vi "OAT Tachless Connect Trace.vi"(10 "Pop Pos":cluster{i32, i32}, 11 "Tracks Ref":refnum<vi>) -> ()   [LabVIEW 2017, in "SoundVib_Tachless.lvlib"]
uses:
  <vilib>/addons/Sound and Vibration/Order Analysis/Tachless/SoundVib_Tachless.lvlib
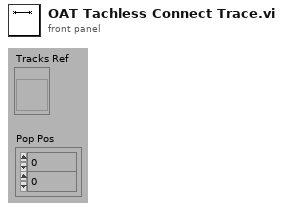
[diagram p1: front panel]
types:
  T1 = cluster{"Name":string, "Color":u32, "Style":u8, "Point Style":u8, "Name Visible":bool, "Allow Drag":bool, "Lock Style":u32, "Plot":u32, "Index":i32, "Position":cluster{"X":dbl, "Y":dbl}}[]
  T2 = cluster{"Name":string, "Color":u32, "Hair Style":u8, "Point Style":u8, "Name Visible":bool, "Trackable":bool, "Lock Style":u32, "Plot Number":u32, "Marker Index":i32, "Location":cluster{"X":dbl, "Y":dbl}}[]
  T3 = cluster{"Name":string, "Color":u32, "Hair Style":u8, "Point Style":u8, "Name Visible":bool, "Trackable":bool, "Lock Style":u32, "Plot Number":u32, "Marker Index":i32, "Location":cluster{"X":dbl, "Y":dbl}}
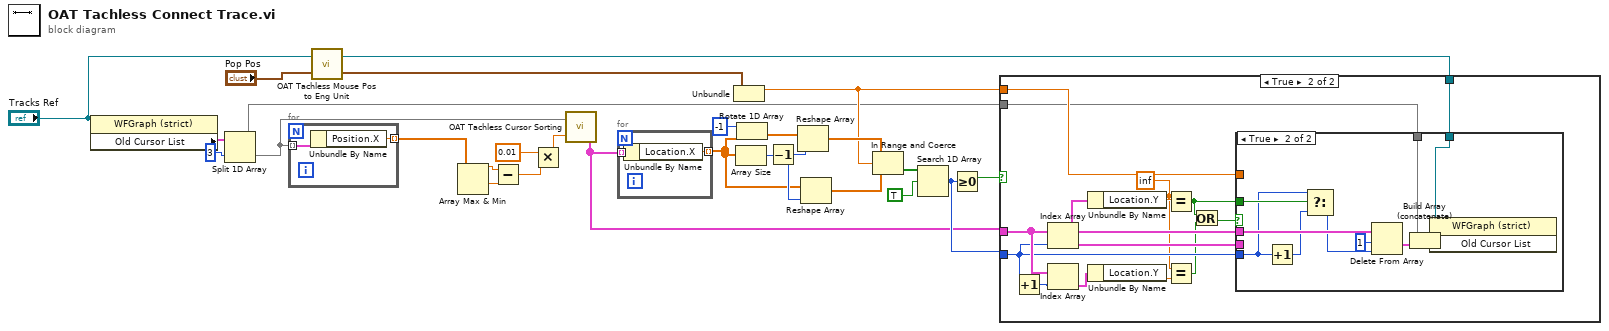
[diagram p0: block diagram]
diagram:
  n1 = property on="Property Node" class="WFGraph (strict)"(reference="Tracks Ref") -> ("Old Cursor List"=w25:T1)  [unwired: 1 in, 2 out]
  n2 = Split 1D Array(array=w25, index=3 ("Array Index")) -> (first subarray=w3:T1, second subarray=w2:T1)
  n3 = for {
    tunnel: w2 -> [w28] mode=indexing
    tunnel: [w27] -> w5 mode=indexing
    n4 = Unbundle By Name(w28) -> ("Position.X"=w27:dbl)
  }
  n5 = call <vilib>:"OAT Tachless Mouse Pos to Eng Unit.vi"("Pop Pos"="Pop Pos", "Tracks ref"="Tracks Ref") -> ("Control Point"=w17:cluster{dbl, dbl})  [unwired: 1 in]
  n6 = Array Max & Min(array=w5) -> (max value=w10:dbl, min value=w9:dbl)  [unwired: 2 out]
  n7 = Subtract(x=w10, y=w9) -> (x-y=w8:dbl)
  n8 = Multiply(x=0.01, y=w8) -> (x*y=w6:dbl)
  n9 = call <vilib>:"OAT Tachless Cursor Sorting.vi"("Numeric"=w6, "Array"=w2) -> ("Array 2"=w1:T2)
  n10 = for {
    tunnel: w1 -> [w30] mode=indexing
    tunnel: [w29] -> w4 mode=indexing
    n11 = Unbundle By Name(w30) -> ("Location.X"=w29:dbl)
  }
  n12 = Unbundle(w17) -> (w14:dbl)  [unwired: 1 out]
  n13 = Array Size(array=w4) -> (size(s)=w21:i32)
  n14 = Rotate 1D Array(1:w4, 2:-1 ("n")) -> (0:w22:dbl[])
  n15 = Decrement(x=w21) -> (x-1=w20:i32)
  n16 = Reshape Array(w22, w20) -> (w19:dbl[])
  n17 = Reshape Array(w4, w20) -> (w18:dbl[])
  n18 = In Range and Coerce(upper limit=w19, x=w14, lower limit=w18) -> (In Range?=w16:bool[])  [unwired: 1 out]
  n19 = Search 1D Array(1D array=w16, element=TRUE) -> (index of element=w13:i32)  [unwired: 1 in]
  n20 = Greater Or Equal To 0?(x=w13) -> (x >= 0?=w12:bool)
  n21 = case shown="True" w12 {
    tunnel: w13 -> [_ w39]
    tunnel: w1 -> [_ w40]
    tunnel: w14 -> [_ w43]
    tunnel: "Tracks Ref" -> [_ w42]
    tunnel: w3 -> [_ w41]
    frame False {
    }
    frame True {
      w31 = inf ("x")
      n22 = Increment(x=w39) -> (x+1=w38:i32)
      n23 = Index Array(array=w40, index=w39) -> (element=w44:T3)
      n24 = Index Array(array=w40, index=w38) -> (element=w37:T3)
      n25 = Unbundle By Name(w44) -> ("Location.Y"=w36:dbl)
      n26 = Unbundle By Name(w37) -> ("Location.Y"=w35:dbl)
      n27 = Equal?(x=w31, y=w36) -> (x = y?=w34:bool)
      n28 = Equal?(x=w31, y=w35) -> (x = y?=w33:bool)
      n29 = Or(x=w34, y=w33) -> (x .or. y?=w32:bool)
      n30 = case shown="True" w32 {
        tunnel: w44 -> [_ _]
        tunnel: w43 -> [_ _]
        tunnel: w42 -> [_ w53]
        tunnel: w41 -> [_ w51]
        tunnel: w40 -> [_ w50]
        tunnel: w39 -> [_ w48]
        tunnel: w34 -> [_ w49]
        frame False {
        }
        frame True {
          n31 = Increment(x=w48) -> (x+1=w46:i32)
          n32 = Select(t=w48, s=w49, f=w46) -> (s? t:f=w45:i32)
          n33 = Delete From Array(array=w50, length=1 ("Length"), index=w45) -> (array with subset deleted=w54:T2)  [unwired: 1 out]
          n34 = Build Array (concatenate)(w51, w54) -> (w52:T2)
          n35 = property on="Property Node" class="WFGraph (strict)"(reference=w53, "Old Cursor List"=w52) -> ()  [unwired: 1 in, 2 out]
        }
      }
    }
  }
